vi "Write Measurement Function Ring.vi"(8 "error in (no error)":errorcluster, 10 "Strings And Values []":T1, 11 "Generic Digital Multi Meter in":refnum<class "Generic Digital Multi Meter.lvclass">) -> (0 "error out":errorcluster, 3 "Generic Digital Multi Meter out":refnum<class "Generic Digital Multi Meter.lvclass">)   [LabVIEW 2014, in "Generic Digital Multi Meter.lvlib" / "Generic Digital Multi Meter.lvclass"]
uses:
  Generic Digital Multi Meter.lvclass
  <vilib>/Utility/miscctls.llb/LVStringsAndValuesArrayTypeDef_U16.ctl
  Generic Digital Multi Meter.lvclass/Generic Digital Multi Meter.ctl
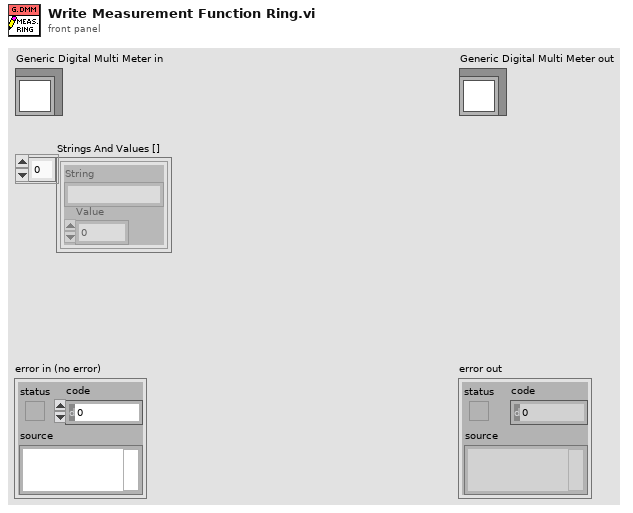
[diagram p1: front panel]
types:
  T1 = typedef "LVStringsAndValuesArrayTypeDef_U16.ctl" = cluster{"String":string, "Value":u16}[]
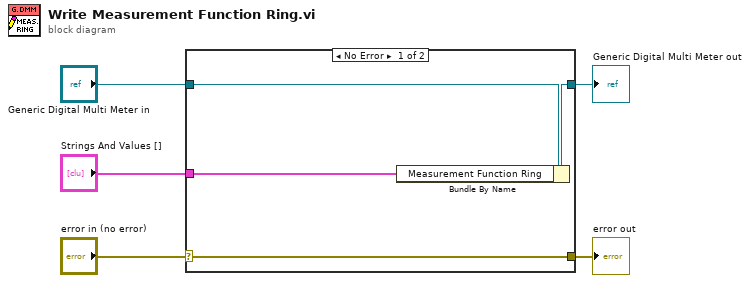
[diagram p0: block diagram]
diagram:
  n1 = case shown="No Error" "error in (no error)" {
    selector: "error in (no error)" -> [w9 w10]
    tunnel: [w9 w10] -> w4
    tunnel: [w7 w11] -> w2
    tunnel: "Generic Digital Multi Meter in" -> [w8 w11]
    tunnel: "Strings And Values []" -> [w6 _]
    frame No Error {
      n2 = Bundle By Name(cluster=w8, "Measurement Function Ring"=w6) -> (w7:refnum<class "Generic Digital Multi Meter.lvclass">)
    }
    frame Error {
    }
  }
  "error out" <- w4
  "Generic Digital Multi Meter out" <- w2
